vi "6_Using_LabVIEW_native_Digital_and_Analog_Waveform.vi"() -> ()   [LabVIEW 2014]
doc: "This example illustrates how the use of the Digital Data controls and how to construct a Digital Waveform from individual components. A Digital Waveform Graph represents the signals graphically. Attention is placed on the distinctions of signal versus sample and directions are given on displaying the plots in the form of a single bus or individually."
uses:
  <vilib>/Swabian Instruments/Pulse Streamer/PulseStreamer/PulseStreamer/stream/stream (Sequence).vi
  <vilib>/Swabian Instruments/Pulse Streamer/PulseStreamer/PulseStreamer.lvlib
  <vilib>/Swabian Instruments/Pulse Streamer/PulseStreamer/PulseStreamer/PulseStreamer.lvclass
panel:
  in  "n_runs":i64=-1
  out "Waveform Graph":waveform(dbl)(graph)
  in  "ip or hostname":string="pulsestreamer"
  out "sine waveform":waveform(dbl)={"t0"=timestamp(0 s since 1904-01-01), "dt"=100.0, "Y"=[0.0, 0.6427876096865393, 0.984807753012208, 0.8660254037844387, 0.3420201433256689, -0.34202014332566866, -0.8660254037844384, -0.9848077530122081, -0.6427876096865396]}
  in  "delta t":dbl=100.0
  in  "n cycles":dbl=1.0
  in  "n points":i32=9
  in  "amplitude":dbl=1.0 min=-1.0 max=1.0
  in  "error in (no error)":errorcluster
  out "error out":errorcluster
  in  "Digital Data":digitaldata={"transitions"=[], "data"=[[0, 0, 0, 0, 0, 0, 0, 0], [0, 0, 0, 0, 0, 0, 0, 1], [0, 0, 0, 0, 0, 0, 1, 1], [0, 0, 0, 0, 0, 1, 1, 1], [0, 0, 0, 0, 1, 1, 1, 1], [0, 0, 0, 1, 1, 1, 1, 1], [0, 0, 1, 1, 1, 1, 1, 1], [0, 1, 1, 1, 1, 1, 1, 1], [1, 1, 1, 1, 1, 1, 1, 1]]}
  out "Digital Waveform Graph":digitalwaveform(graph)={"t0"=timestamp(0 s since 1904-01-01), "dt"=100.0, "Y"={"transitions"=[], "data"=[[0, 0, 0, 0, 0, 0, 0, 0], [0, 0, 0, 0, 0, 0, 0, 1], [0, 0, 0, 0, 0, 0, 1, 1], [0, 0, 0, 0, 0, 1, 1, 1], [0, 0, 0, 0, 1, 1, 1, 1], [0, 0, 0, 1, 1, 1, 1, 1], [0, 0, 1, 1, 1, 1, 1, 1], [0, 1, 1, 1, 1, 1, 1, 1], [1, 1, 1, 1, 1, 1, 1, 1]]}}
  # "Creates a digital and analog waveform with LabVIEW and converts it into a sequence for the Pulse Streamer in Run Length Encoding (RLE)"
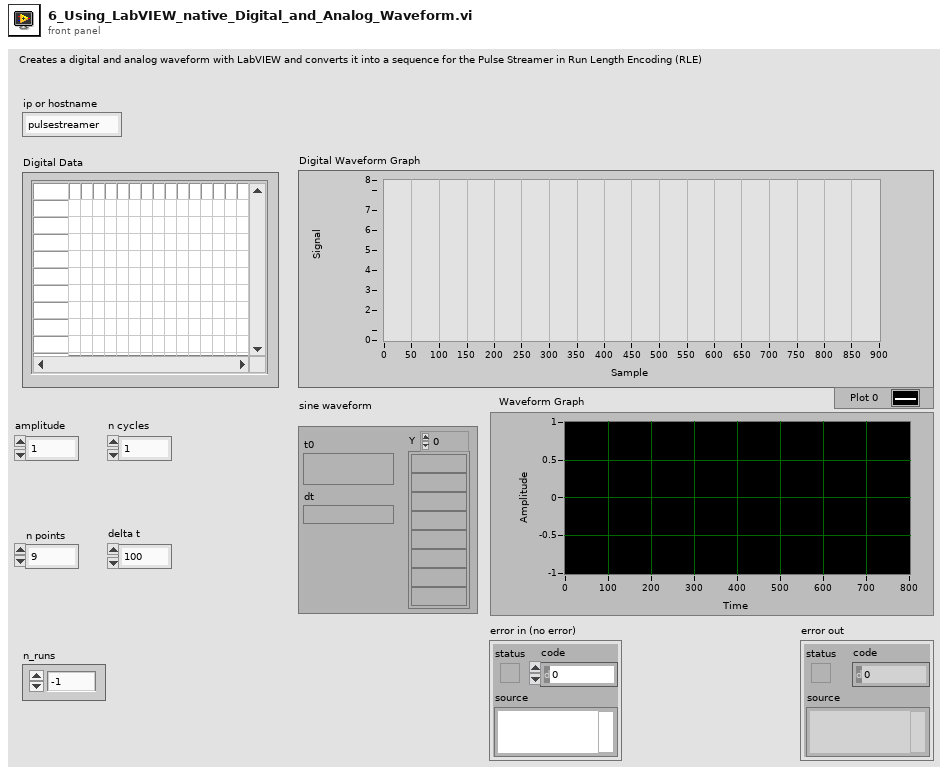
[diagram p1: front panel]
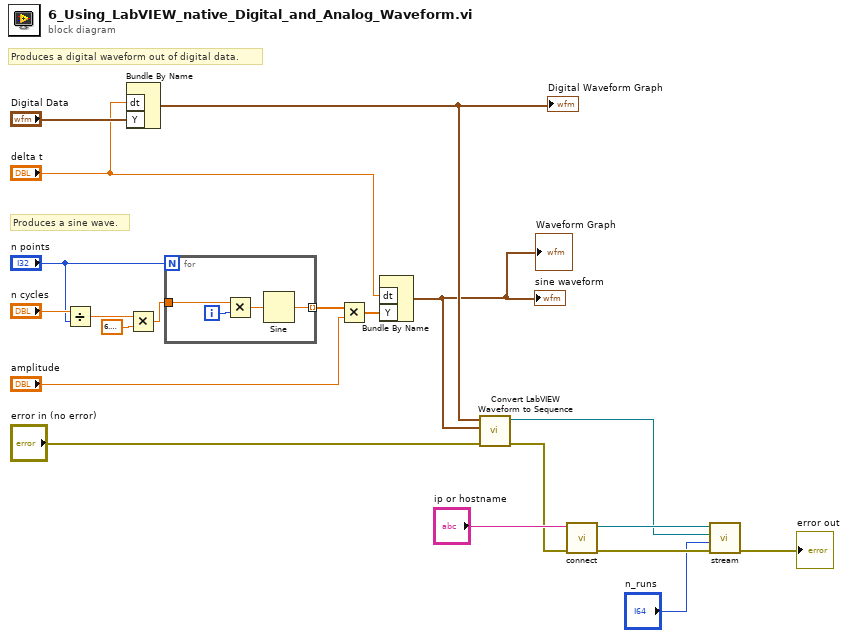
[diagram p0: block diagram]
diagram:
  # "Produces a sine wave."
  # "Produces a digital waveform out of digital data."
  n1 = Divide(x="n cycles", y="n points") -> (x/y=w14:dbl)
  n2 = Bundle By Name("dt"="delta t", "Y"="Digital Data") -> (w19:digitalwaveform)  [unwired: 1 in]
  "Digital Waveform Graph" <- w19
  n3 = Multiply(x=w14, y=6.283185307179586) -> (x*y=w12:dbl)
  n4 = for {
    N: "n points" -> [_]
    tunnel: [w24] -> w17 mode=indexing
    tunnel: w12 -> [w21]
    i -> [w22]
    n5 = Multiply(x=w21, y=w22) -> (x*y=w23:dbl)
    n6 = Sine(x=w23) -> (sin(x)=w24:dbl)
  }
  n7 = Multiply(x=w17, y="amplitude") -> (x*y=w10:dbl[])
  n8 = Bundle By Name("dt"="delta t", "Y"=w10) -> (w3:waveform(dbl))  [unwired: 1 out]
  "sine waveform" <- w3
  "Waveform Graph" <- w3
  n9 = call <vilib>:"Convert LabVIEW Waveform to Sequence.vi"("error in (no error)"="error in (no error)", "Waveform Analog 0"=w3, "Waveform Digital"=w19) -> ("error out"=w7:errorcluster, "Sequence out"=w2:refnum<class "Sequence.lvclass">)  [unwired: 7 in]
  n10 = call <vilib>:"connect.vi"("error in (no error)"=w7, "ip"="ip or hostname") -> ("error out"=w6:errorcluster, "Pulse Streamer out"=w5:refnum<class "PulseStreamer.lvclass">)  [unwired: 8 in]
  n11 = call-poly <vilib>:"stream.vi"("error in (no error)"=w6, "n_runs"="n_runs", "sequence"=w2, "Pulse Streamer in"=w5) -> ("error out"=→"error out":errorcluster)  [unwired: 4 in, 1 out]
